vi "Hello world.vi"() -> ()   [LabVIEW 2020]
panel:
  out "x+y":dbl
  in  "y":dbl
  in  "x":dbl
  in  "Stop":bool
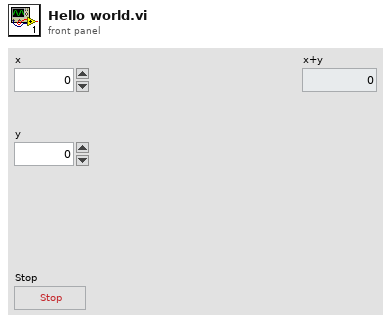
[diagram p1: front panel]
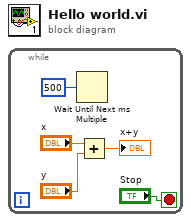
[diagram p0: block diagram]
diagram:
  n1 = while {
    stop <- "Stop" stop-if-true
    n2 = Wait Until Next ms Multiple(millisecond multiple=u32 500) -> ()  [unwired: 1 out]
    n3 = Add(x="x", y="y") -> (x+y=→"x+y":dbl)
  }
